vi "Animate To Focused.vi"(8 "error in (no error)":errorcluster, 11 "Filled Text Fields Actor in":refnum<class "Filled Text Fields Actor.lvclass">) -> (0 "error out":errorcluster, 3 "Filled Text Fields Actor out":refnum<class "Filled Text Fields Actor.lvclass">)   [LabVIEW 2017, in "Filled Text Fields.lvlib" / "Filled Text Fields Actor.lvclass"]
uses:
  Filled Text Fields Actor.lvclass
  Filled Text Fields Actor.lvclass/Filled Text Fields Actor.ctl
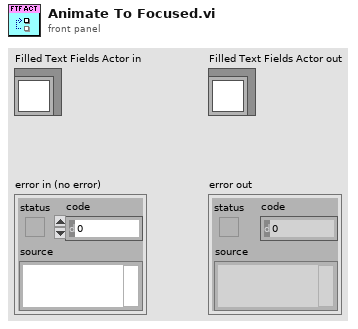
[diagram p1: front panel]
types:
  T1 = typedef "Theme.lvlib/Theme.Font.lvclass/Font.ctl" = cluster{"Size":u32, "Shrink Size":u32, "Name":string, "Password Display":bool}
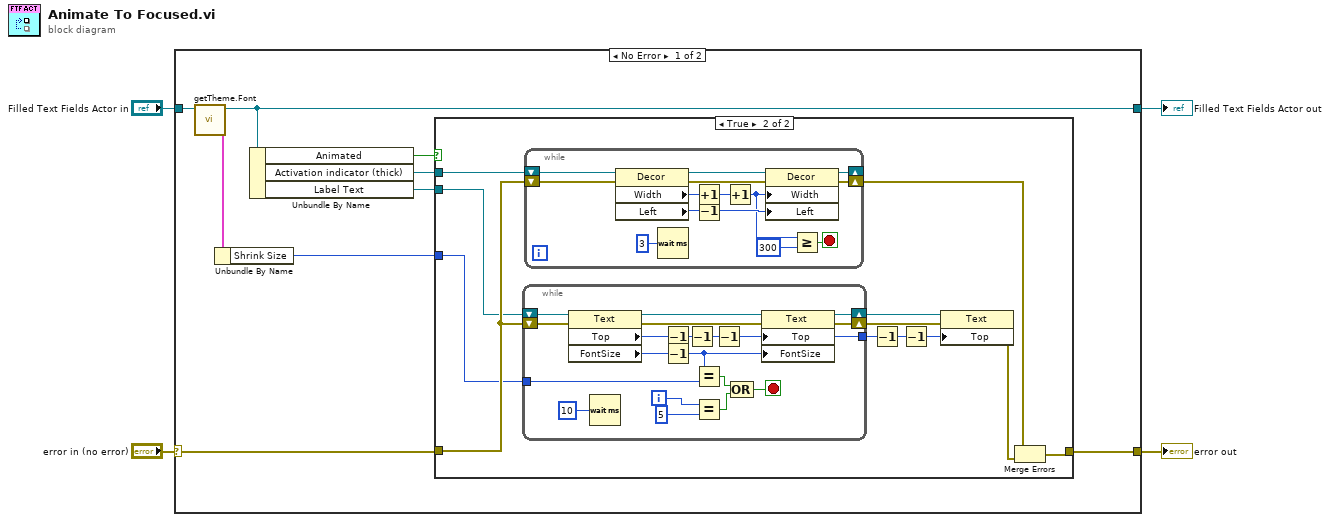
[diagram p0: block diagram]
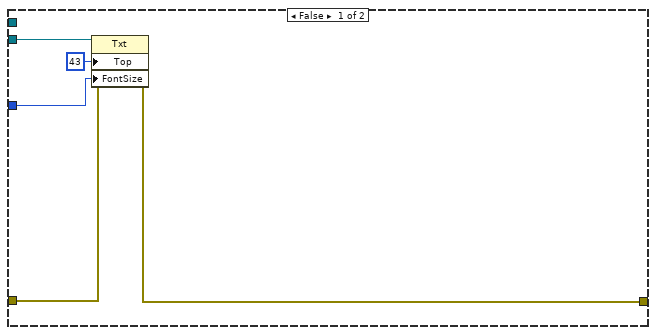
[diagram p2: hidden frame]
diagram:
  n1 = case shown="No Error" "error in (no error)" {
    selector: "error in (no error)" -> [w9 w65]
    tunnel: [w8 w65] -> w3
    tunnel: [w7 w64] -> w1
    tunnel: "Filled Text Fields Actor in" -> [w13 w64]
    frame No Error {
      n2 = call "getTheme.Font.vi"("Filled Text Fields Actor in"=w13) -> ("Font"=w6:T1, "Filled Text Fields Actor out"=w7:refnum<class "Filled Text Fields Actor.lvclass">)  [unwired: 9 in]
      n3 = Unbundle By Name(w6) -> ("Shrink Size"=w5:u32)
      n4 = Unbundle By Name(w7) -> ("Animated"=w12:bool, "Activation indicator (thick)"=w11:refnum<vi>, "Label Text"=w10:refnum<vi>)
      n5 = case shown="True" w12 {
        tunnel: w11 -> [_ w21]
        tunnel: w10 -> [w15 w20]
        tunnel: w9 -> [w17 w24]
        tunnel: [w16 w23] -> w8
        tunnel: w5 -> [w14 w19]
        frame False {
          n6 = property class="Txt"(reference=w15, error in=w17, "Top"=43 ("Position:Top"), "FontSize"=w14) -> (error out=w16:errorcluster)  [unwired: 1 out]
        }
        frame True {
          n7 = while {
            shift-right: [w58] -> w30
            shift-left: w20 -> [w57]
            tunnel: [w54] -> w27
            shift-right: [w48] -> w26
            shift-left: w24 -> [w46]
            tunnel: w19 -> [w45]
            i -> [w53]
            stop <- w49 stop-if-true
            n8 = property on="Property Node" class="Text"(reference=w57, error in=w46) -> (reference out=w62:refnum<vi>, error out=w47:errorcluster, "Top"=w60:i32, "FontSize"=w59:u32)
            n9 = Wait (ms)(milliseconds to wait=u32 10) -> ()  [unwired: 1 out]
            n10 = Decrement(x=w60) -> (x-1=w56:i32)
            n11 = Decrement(x=w59) -> (x-1=w63:u32)
            n12 = Decrement(x=w56) -> (x-1=w55:i32)
            n13 = Equal?(x=w63, y=w45) -> (x = y?=w51:bool)
            n14 = Equal?(x=w53, y=5) -> (x = y?=w50:bool)
            n15 = Decrement(x=w55) -> (x-1=w54:i32)
            n16 = Compound Arithmetic op=OR(w51, w50) -> (w49:bool)
            n17 = property on="Property Node" class="Text"(reference=w62, error in=w47, "Top"=w54, "FontSize"=w63) -> (reference out=w58:refnum<vi>, error out=w48:errorcluster)
          }
          n18 = while {
            shift-right: [w35] -> _
            shift-left: w21 -> [w34]
            shift-right: [w32] -> w22
            shift-left: w24 -> [w31]
            stop <- w43 stop-if-true
            n19 = property class="Decor"(reference=w34, error in=w31) -> (reference out=w38:refnum<vi>, error out=w33:errorcluster, "Width"=w41:u32, "Left"=w40:i32)
            n20 = Wait (ms)(milliseconds to wait=u32 3) -> ()  [unwired: 1 out]
            n21 = Increment(x=w41) -> (x+1=w37:u32)
            n22 = Decrement(x=w40) -> (x-1=w39:i32)
            n23 = Increment(x=w37) -> (x+1=w36:u32)
            n24 = property class="Decor"(reference=w38, error in=w33, "Width"=w36, "Left"=w39) -> (reference out=w35:refnum<vi>, error out=w32:errorcluster)
            n25 = Greater Or Equal?(x=w36, y=u32 300 ("Deco Width Max")) -> (x >= y?=w43:bool)
          }
          n26 = Decrement(x=w27) -> (x-1=w28:i32)
          n27 = Decrement(x=w28) -> (x-1=w29:i32)
          n28 = property on="Property Node" class="Text"(reference=w30, error in=w26, "Top"=w29) -> (error out=w25:errorcluster)  [unwired: 1 out]
          n29 = Merge Errors(w22, w25) -> (w23:errorcluster)
        }
      }
    }
    frame Error {
    }
  }
  "error out" <- w3
  "Filled Text Fields Actor out" <- w1
